vi "PKG_IMC_SetADCtrlEX.vi"(1 "id":i32, 4 "tgid":i32, 5 "tgEnd":dbl, 6 "tgStart":dbl, 7 "ch":i32, 9 "ADend":dbl, 10 "ADstart":dbl, 11 "handle":u32) -> (2 "function return":i32, 3 "handle out":u32)   [LabVIEW 2011, in "IMC_Pkg4xxx.lvlib"]
doc: "PKG_IMC_SetADCtrlEX(IMC_HANDLE handle, double ADstart, double ADend, int ch, double tgStart, double tgEnd, int tgid, int id);"
uses:
  IMC_Pkg4xxx.lvlib
  IMC_Pkg4xxx.dll
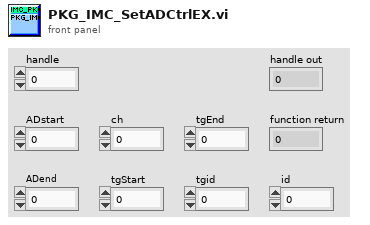
[diagram p1: front panel]
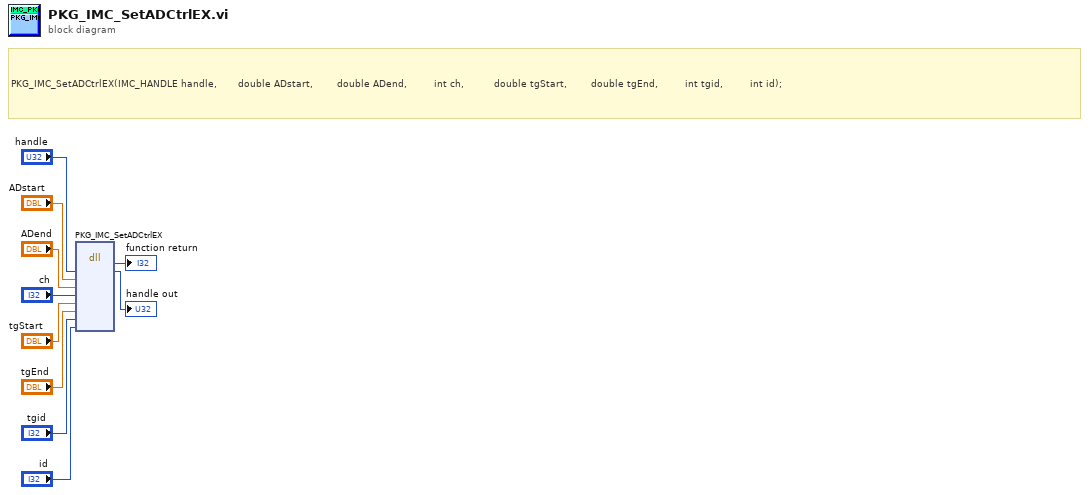
[diagram p0: block diagram]
diagram:
  # "PKG_IMC_SetADCtrlEX(IMC_HANDLE handle,  \t\t\t\t\tdouble ADstart, \t\t\t\t\t\t\tdouble ADend, \t\t\t\t\t\t\t\tint ch, \t\t\t\t\t\t\t\t\tdouble tgStart, \t\t\t\t\t\t\tdouble tgEnd, \t\t\t\t\t\t\t\tint tgid,\t\t\t\t\t\t\t\t\tint id);"
  n1 = dll-call lib="PTH1mabs F光盘刻录\niMC MotionIMCNet_V4.0IMCAppincLabviewIMC_PKG4xxxIMC_PKG4xxx\nIMC_Pkg4xxx.*" fn="PKG_IMC_SetADCtrlEX"("handle"="handle", "ADstart"="ADstart", "ADend"="ADend", "ch"="ch", "tgStart"="tgStart", "tgEnd"="tgEnd", "tgid"="tgid", "id"="id") -> (→"function return":i32, "handle"=→"handle out":u32)  [unwired: 10 in, 2 out]
